vi "Write Experiment Description.vi"(8 "error in (no error)":errorcluster, 10 "Experiment Description":string, 11 "Control Experiment in":refnum<class "Control Experiment.lvclass">) -> (0 "error out":errorcluster, 3 "Control Experiment out":refnum<class "Control Experiment.lvclass">)   [LabVIEW 2019, in "Control Experiment.lvclass"]
uses:
  Control Experiment.lvclass
  Control Experiment.lvclass/Control Experiment.ctl
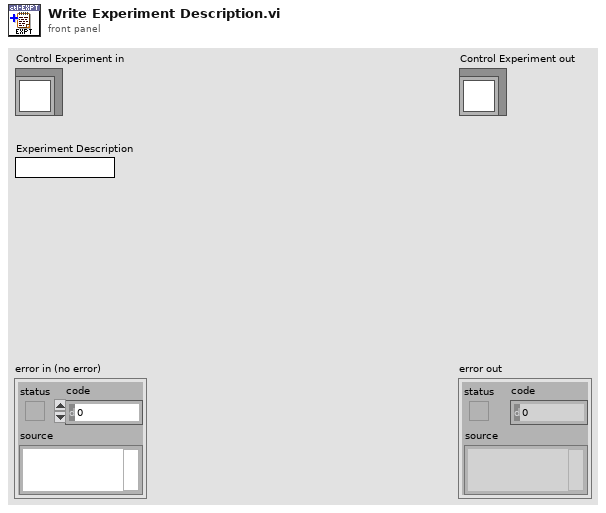
[diagram p1: front panel]
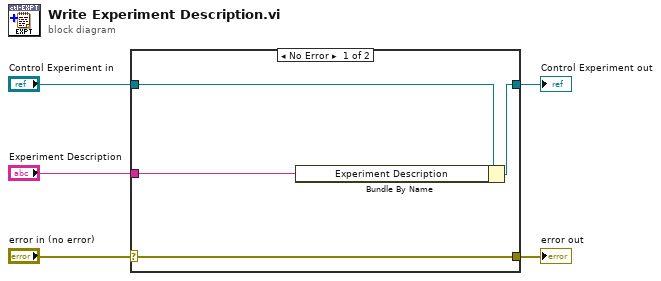
[diagram p0: block diagram]
diagram:
  n1 = case shown="No Error" "error in (no error)" {
    selector: "error in (no error)" -> [w9 w10]
    tunnel: [w9 w10] -> w4
    tunnel: [w7 w11] -> w2
    tunnel: "Control Experiment in" -> [w8 w11]
    tunnel: "Experiment Description" -> [w6 _]
    frame No Error {
      n2 = Bundle By Name(cluster=w8, "Experiment Description"=w6) -> (w7:refnum<class "Control Experiment.lvclass">)
    }
    frame Error {
    }
  }
  "error out" <- w4
  "Control Experiment out" <- w2
